vi "Dictionary to Chart.vi"(6 "History Length [1024]":i32=1024, 7 "reset":bool, 8 "error in (no error)":errorcluster, 10 "Fs.Output (S/s)":dbl, 11 "Results (Dictionary)":cluster{"key":string, "value":dbl[]}[](array[cluster])) -> (0 "error out":errorcluster, 2 "Waveform Graph":waveform(dbl)[][](array[waveform]), 3 "Results (Dictionary) out":cluster{"key":string, "value":dbl[]}[](array[cluster]))   [LabVIEW 2019, in "Instrument.Lockin.lvlib" / "Instrument UI.Lockin.lvclass"]
uses:
  Instrument UI.Lockin.lvclass
  Instrument.Lockin/Typedefs/Results Type--Enum.ctl
  <vilib>/PRIrvin/XY Utilities/subVIs/Circular Buffer (waveforms).vi
  Instrument.Lockin/Instrument.Lockin.lvclass
  <vilib>/PRIrvin/XY Utilities/xy_utilities.lvlib
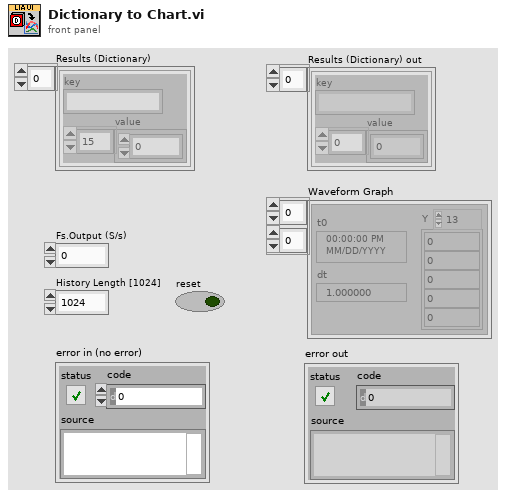
[diagram p1: front panel]
types:
  T1 = typedef "Instrument.Lockin.lvlib/Instrument.Lockin.lvclass/Results Type--Enum.ctl" = enum16{"X", "Y", "R", "Theta", "Mean"}
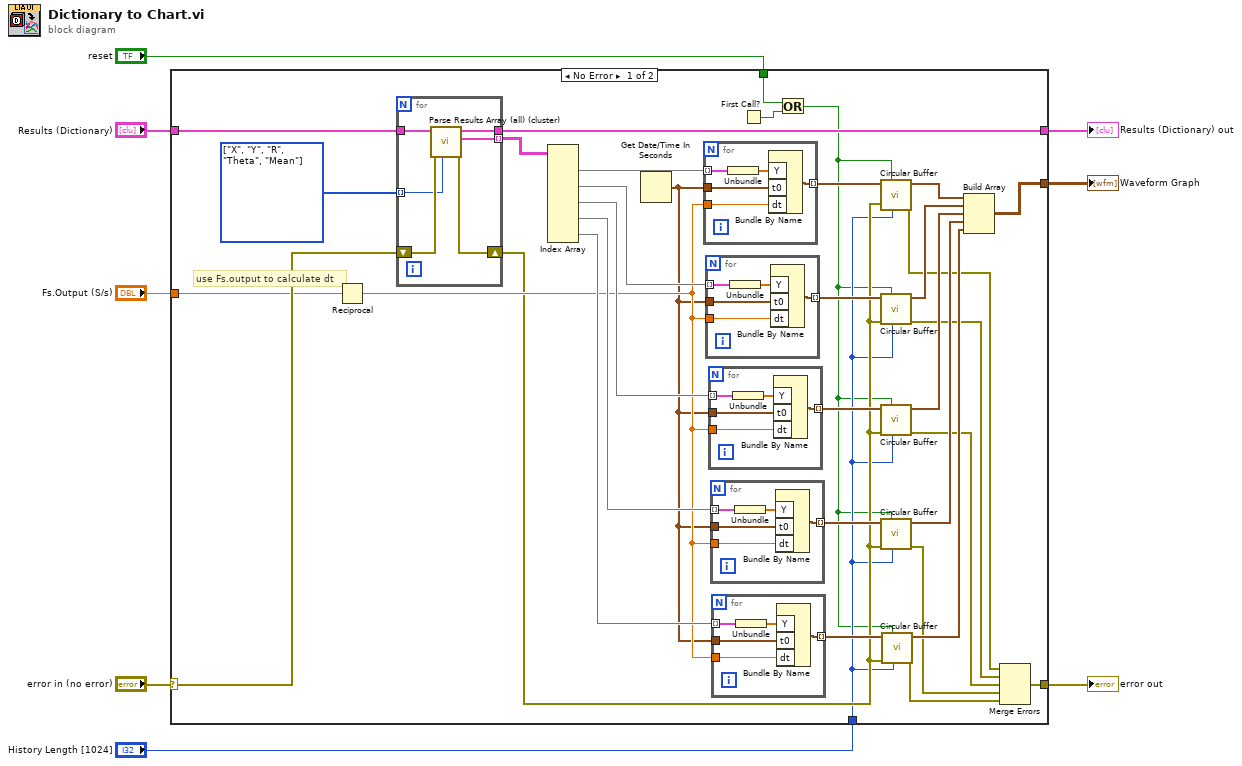
[diagram p0: block diagram]
diagram:
  n1 = case shown="No Error" "error in (no error)" {
    selector: "error in (no error)" -> [w42 w76]
    tunnel: [w22 _] -> w8
    tunnel: "Results (Dictionary)" -> [w43 w75]
    tunnel: [w18 w76] -> w5
    tunnel: [w41 w75] -> w4
    tunnel: "Fs.Output (S/s)" -> [w40 _]
    tunnel: "reset" -> [w10 _]
    tunnel: "History Length [1024]" -> [w12 _]
    frame No Error {
      w39 = T1[] [enum."X", enum."Y", enum."R", enum."Theta", enum."Mean"] items=["X", "Y", "R", "Theta", "Mean"] ("Array")
      # "use Fs.output to calculate dt"
      n2 = Reciprocal(x=w40) -> (1/x=w21:dbl)
      n3 = for {
        tunnel: w43 -> [w74]
        tunnel: [w72] -> w41
        tunnel: w39 -> [w71] mode=indexing
        tunnel: [w69] -> w36 mode=indexing
        shift-right: [w70] -> w19
        shift-left: w42 -> [w73]
        n4 = call "Parse Results Array (all) (cluster).vi"("Type"=w71, "error in (no error)"=w73, "Results (Dictionary)"=w74) -> ("error out"=w70:errorcluster, "Data"=w69:cluster{"value":dbl[]}[], "Results (Dictionary)"=w72:cluster{"key":string, "value":dbl[]}[])  [unwired: 5 in, 1 out]
      }
      n5 = Index Array(array=w36) -> (element #1=w37:cluster{"value":dbl[]}[], element #2=w31:cluster{"value":dbl[]}[], element #3=w30:cluster{"value":dbl[]}[], element #4=w29:cluster{"value":dbl[]}[], element #5=w28:cluster{"value":dbl[]}[])  [unwired: 10 in]
      n6 = Get Date/Time In Seconds() -> (seconds since 1Jan1904=w20:timestamp)
      n7 = for {
        tunnel: w37 -> [w67] mode=indexing
        tunnel: [w68] -> w38 mode=indexing
        tunnel: w20 -> [w66]
        tunnel: w21 -> [w64]
        n8 = Unbundle(w67) -> ("value"=w65:dbl[])
        n9 = Bundle By Name("Y"=w65, "t0"=w66, "dt"=w64) -> (w68:waveform(dbl))  [unwired: 1 in]
      }
      n10 = for {
        tunnel: w31 -> [w62] mode=indexing
        tunnel: [w63] -> w35 mode=indexing
        tunnel: w20 -> [w61]
        tunnel: w21 -> [w59]
        n11 = Unbundle(w62) -> ("value"=w60:dbl[])
        n12 = Bundle By Name("Y"=w60, "t0"=w61, "dt"=w59) -> (w63:waveform(dbl))  [unwired: 1 in]
      }
      n13 = for {
        tunnel: w30 -> [w57] mode=indexing
        tunnel: [w58] -> w33 mode=indexing
        tunnel: w20 -> [w56]
        tunnel: w21 -> [w54]
        n14 = Unbundle(w57) -> ("value"=w55:dbl[])
        n15 = Bundle By Name("Y"=w55, "t0"=w56, "dt"=w54) -> (w58:waveform(dbl))  [unwired: 1 in]
      }
      n16 = for {
        tunnel: w29 -> [w52] mode=indexing
        tunnel: [w53] -> w34 mode=indexing
        tunnel: w20 -> [w51]
        tunnel: w21 -> [w49]
        n17 = Unbundle(w52) -> ("value"=w50:dbl[])
        n18 = Bundle By Name("Y"=w50, "t0"=w51, "dt"=w49) -> (w53:waveform(dbl))  [unwired: 1 in]
      }
      n19 = for {
        tunnel: w28 -> [w47] mode=indexing
        tunnel: [w48] -> w32 mode=indexing
        tunnel: w20 -> [w46]
        tunnel: w21 -> [w44]
        n20 = Unbundle(w47) -> ("value"=w45:dbl[])
        n21 = Bundle By Name("Y"=w45, "t0"=w46, "dt"=w44) -> (w48:waveform(dbl))  [unwired: 1 in]
      }
      n22 = First Call?() -> (First Call?: T/F=w9:bool)
      n23 = Or(x=w10, y=w9) -> (x .or. y?=w11:bool)
      n24 = call-poly <vilib>:"Circular Buffer.vi"("History Length [1024]"=w12, "reset"=w11, "error in"=w19, "Waveform in"=w38) -> ("error out"=w13:errorcluster, "Waveform out"=w23:waveform(dbl)[])  [unwired: 6 in]
      n25 = call-poly <vilib>:"Circular Buffer.vi"("History Length [1024]"=w12, "reset"=w11, "error in"=w19, "Waveform in"=w35) -> ("error out"=w14:errorcluster, "Waveform out"=w24:waveform(dbl)[])  [unwired: 6 in]
      n26 = call-poly <vilib>:"Circular Buffer.vi"("History Length [1024]"=w12, "reset"=w11, "error in"=w19, "Waveform in"=w33) -> ("error out"=w15:errorcluster, "Waveform out"=w25:waveform(dbl)[])  [unwired: 6 in]
      n27 = call-poly <vilib>:"Circular Buffer.vi"("History Length [1024]"=w12, "reset"=w11, "error in"=w19, "Waveform in"=w34) -> ("error out"=w16:errorcluster, "Waveform out"=w26:waveform(dbl)[])  [unwired: 6 in]
      n28 = call-poly <vilib>:"Circular Buffer.vi"("History Length [1024]"=w12, "reset"=w11, "error in"=w19, "Waveform in"=w32) -> ("error out"=w17:errorcluster, "Waveform out"=w27:waveform(dbl)[])  [unwired: 6 in]
      n29 = Build Array(w23, w24, w25, w26, w27) -> (w22:waveform(dbl)[][])
      n30 = Merge Errors(w13, w14, w15, w16, w17) -> (w18:errorcluster)
    }
    frame Error {
    }
  }
  "Waveform Graph" <- w8
  "error out" <- w5
  "Results (Dictionary) out" <- w4
